vi "TL behavior get unstuck_D2.vi"(2 "Behavior\nVelocity":dbl, 3 "Activate?":bool=TRUE, 4 "Numeric":dbl, 5 "Sensor":T1=[{"Name"="bow", "Angle"=20.0, "Distance"=0.0}, {"Name"="pbow", "Angle"=60.0, "Distance"=0.0}, {"Name"="port", "Angle"=0.0, "Distance"=0.0}, {"Name"="sbow", "Angle"=60.0, "Distance"=0.0}, {"Name"="starboard", "Angle"=0.0, "Distance"=0.0}]) -> (0 "Unstuck Array":dbl[](array[numeric]), 1 "Numeric 2":dbl)   [LabVIEW 2014]
uses:
  sensorsSTD.ctl
panel:
  out "Waveform Graph":cluster{dbl, dbl, dbl[]}(graph)
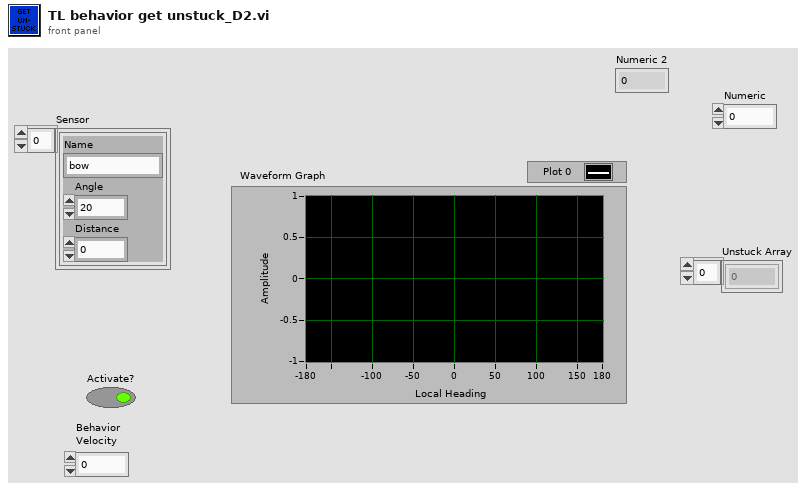
[diagram p1: front panel]
types:
  T1 = typedef "sensorsSTD.ctl" = cluster{"Name":string, "Angle":dbl, "Distance":dbl}[]
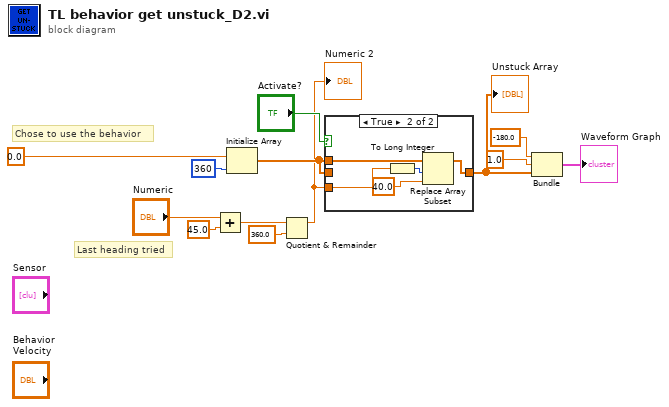
[diagram p0: block diagram]
diagram:
  # "Last heading tried"
  # "Chose to use the behavior"
  n1 = Add(x="Numeric", y=45.0 ("std (Normal)")) -> (x+y=w5:dbl)
  n2 = Initialize Array(0.0 ("element"), 360 ("dimension size")) -> (w7:dbl[])
  n3 = Quotient & Remainder(x=w5, y=360.0 ("std (Normal)")) -> (x-y*floor(x/y)=w1:dbl)  [unwired: 1 out]
  "Numeric 2" <- w1
  n4 = case shown="True" "Activate?" {
    tunnel: w7 -> [w14 _]
    tunnel: w7 -> [_ w19]
    tunnel: [w14 w18] -> w6
    tunnel: w1 -> [_ w16]
    frame False {
    }
    frame True {
      n5 = To Long Integer(number=w16) -> (32bit integer=w15:i32)
      n6 = Replace Array Subset(array=w19, new element=40.0 ("index"), index=w15) -> (w18:dbl[])
    }
  }
  "Unstuck Array" <- w6
  n7 = Bundle(-180.0, 1.0, w6) -> (→"Waveform Graph":cluster{dbl, dbl, dbl[]})  [unwired: 1 in]
